vi "kvCanReadErrorCounters.vi"(0 "Channel Handle (input only)":i32, 1 "error in (no error)":errorcluster) -> (2 "error out":errorcluster, 3 "Channel Handle (ouput only)":i32, 4 "Transmit Errors":u32, 5 "Receive Errors":u32, 6 "Overrun Errors":u32)   [LabVIEW 2022 SP3]
doc: "Reads the error counters of the CAN controller. \n\nNote: canReadErrorCounters returns the latest known values of the error counters in the specified circuit. If the error counters change values precisely when canReadErrorCounters is called, it may not be reflected in the returned result. \n\nNote: Not all CAN controllers provide access to the error counters; in this case, an educated guess is returned."
uses:
  canlib32.dll
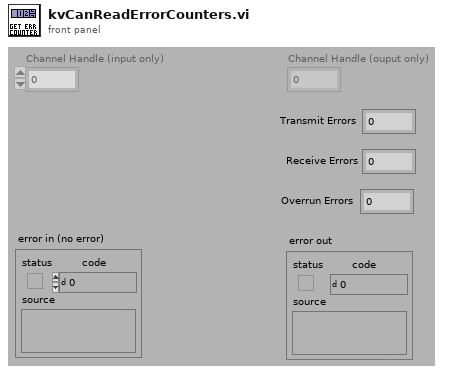
[diagram p1: front panel]
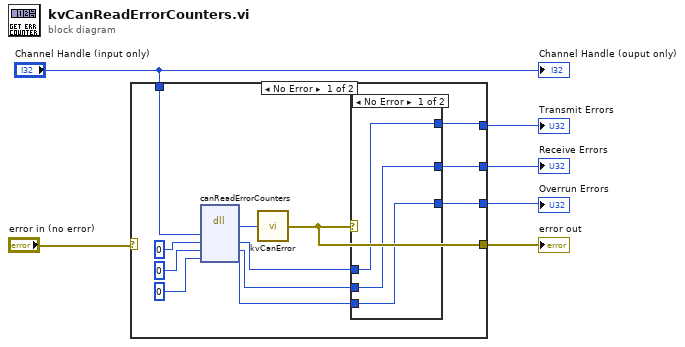
[diagram p0: block diagram]
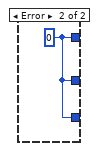
[diagram p2: hidden frame]
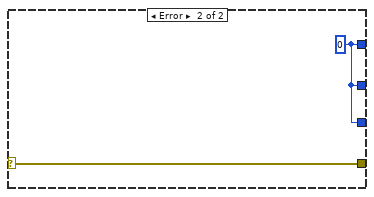
[diagram p3: hidden frame]
diagram:
  n1 = case shown="No Error" "error in (no error)" {
    selector: "error in (no error)" -> [_ w24]
    tunnel: [w10 w24] -> w5
    tunnel: [w13 w23] -> w4
    tunnel: [w12 w23] -> w3
    tunnel: [w11 w23] -> w2
    tunnel: "Channel Handle (input only)" -> [w18 _]
    frame No Error {
      n2 = dll-call lib="canlib32.dll" fn="canReadErrorCounters"("handle"=w18, "txErr"=u32 0, "rxErr"=u32 0, "ovErr"=u32 0) -> (w14:i32, "txErr"=w7:u32, "rxErr"=w8:u32, "ovErr"=w9:u32)  [unwired: 4 in, 2 out]
      n3 = call "kvCanError.vi"("error code"=w14) -> ("error out"=w10:errorcluster)
      n4 = case shown="No Error" w10 {
        tunnel: [w21 w22] -> w13
        tunnel: [w20 w22] -> w12
        tunnel: [w19 w22] -> w11
        tunnel: w9 -> [w19 _]
        tunnel: w8 -> [w20 _]
        tunnel: w7 -> [w21 _]
        frame No Error {
        }
        frame Error {
          w22 = u32 0
        }
      }
    }
    frame Error {
      w23 = u32 0
    }
  }
  "error out" <- w5
  "Transmit Errors" <- w4
  "Receive Errors" <- w3
  "Overrun Errors" <- w2
  "Channel Handle (ouput only)" <- "Channel Handle (input only)"
